vi "GEOM_ReadModifiers.vi"(7 "database path":path, 8 "error in (no error)":errorcluster, 11 "fpa file":path) -> (0 "error out":errorcluster, 2 "modifiers":T2={"Binning"={"x"=1, "y"=1}, "sections"=[]} {"Binning"."y" min=1; "Binning"."x" min=1})   [LabVIEW 2016]
uses:
  GEOM_AmpModifiers.ctl
  GEOM_Binning.ctl
  GEOM_Moifier.ctl
  <vilib>/Utility/config.llb/Read Key (String).vi
  <vilib>/Utility/config.llb/NI_LVConfig.lvlib
panel:
  in  "section":T1
  out "stripped path":path
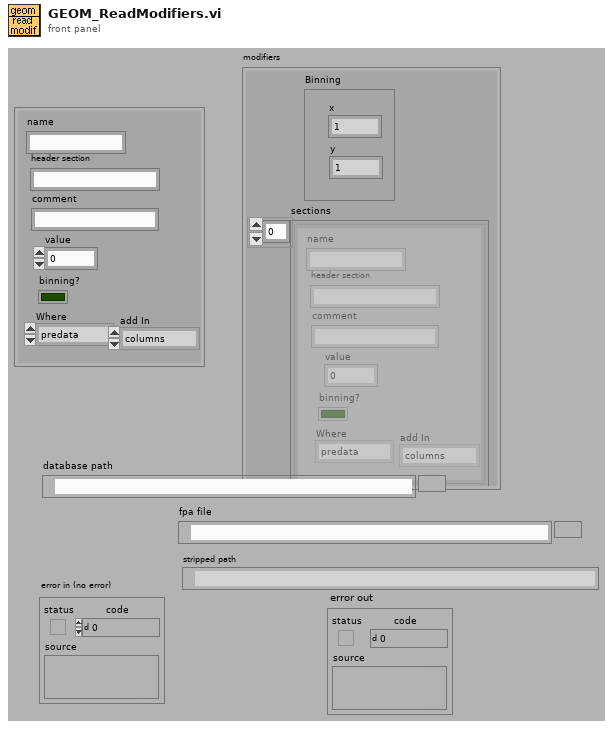
[diagram p1: front panel]
types:
  T1 = cluster{"name":string, "header section":string, "comment":string, "value":i32, "binning?":bool, "Where":enum16{"predata", "postdata"}, "add In":enum16{"columns", "rows", "none"}}
  T2 = typedef "GEOM_AmpModifiers.ctl" = cluster{"Binning":T3, "sections":T4[]}
  T3 = typedef "GEOM_Binning.ctl" = cluster{"x":u32, "y":u32}
  T4 = typedef "GEOM_Moifier.ctl" = cluster{"name":string, "header section":string, "comment":string, "value":i32, "binning?":bool, "Where":enum16{"predata", "postdata"}, "add In":enum16{"columns", "rows", "none"}}
  T5 = cluster{"name":string, "header section":string, "comment":string, "value":i32, "binning?":bool, "Where":enum16{"predata", "postdata"}, "add In":enum16{"columns", "rows", "none"}}[]
  T6 = typedef "NI_LVConfig.lvlib/Config Data RefNum.ctl" = refnum<k1>
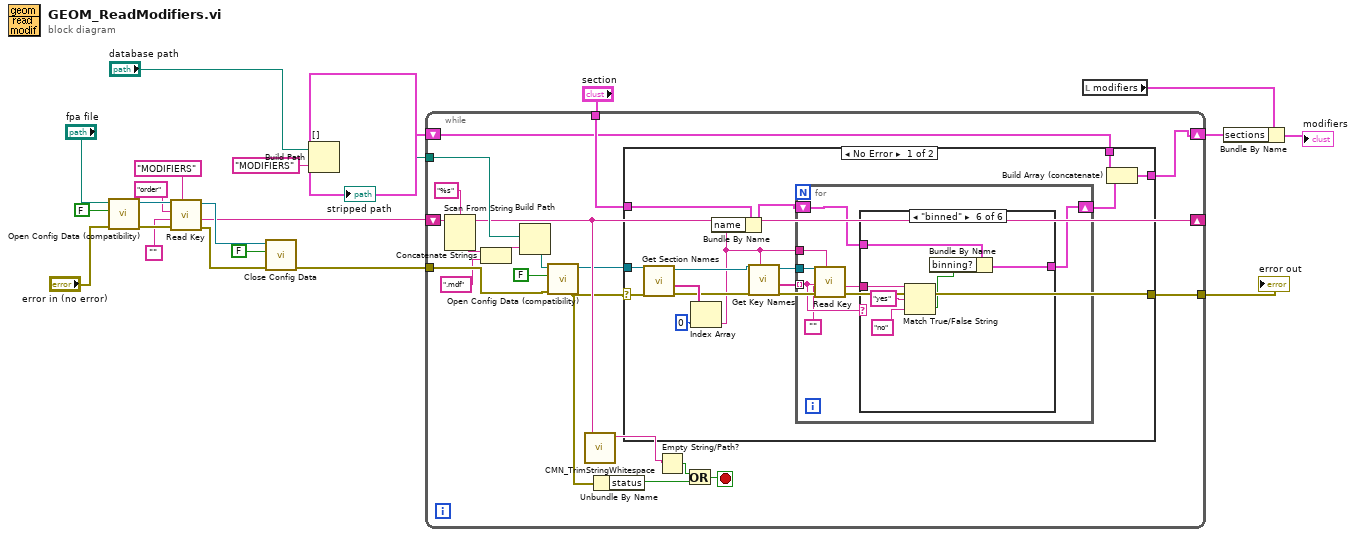
[diagram p0: block diagram]
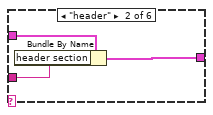
[diagram p3: hidden frame]
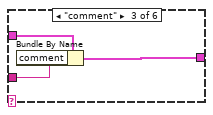
[diagram p4: hidden frame]
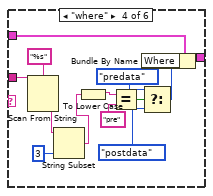
[diagram p5: hidden frame]
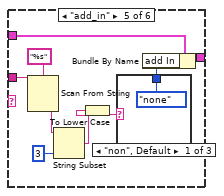
[diagram p6: hidden frame]
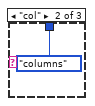
[diagram p7: hidden frame]
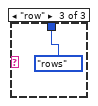
[diagram p8: hidden frame]
diagram:
  n1 = call <vilib>:"Open Config Data (compatibility).vi"("error in (no error)"="error in (no error)", "create file if necessary (T)"=FALSE ("create file if necessary? (T)"), "configuration file path"="fpa file") -> ("error out"=w22:errorcluster, "refnum"=w21:T6)  [unwired: 6 in, 1 out]
  n2 = call-poly <vilib>:"Read Key.vi"("section"="MODIFIERS", "error in (no error)"=w22, "default value"="", "key"="order", "refnum"=w21) -> ("error out"=w16:errorcluster, "value"=w12:string, "refnum out"=w17:T6)  [unwired: 1 in, 3 out]
  n3 = call <vilib>:"Close Config Data.vi"("error in (no error)"=w16, "write file if changed (T)"=FALSE ("write configuration file? (T)"), "refnum"=w17) -> ("error out"=w4:errorcluster)  [unwired: 8 out]
  n4 = Build Path(base path="database path", name or relative path="MODIFIERS") -> (appended path=w11:path)
  "stripped path" <- w11
  n5 = while {
    shift-right: [w37] -> _
    shift-left: w12 -> [w42]
    tunnel: w11 -> [w40]
    tunnel: "section" -> [w31]
    shift-right: [w30] -> w8
    shift-left: T5 [] -> [w29]
    tunnel: w4 -> [w27]
    tunnel: [w26] -> w3
    stop <- w34 stop-if-true
    n6 = Scan From String(format string="%s", input string=w42) -> (remaining string=w37:string, output 1=w25:string)  [unwired: 2 in, 3 out]
    n7 = Concatenate Strings(w25, ".mdf" ("string")) -> (w23:string)
    n8 = Build Path(base path=w40, name or relative path=w23) -> (appended path=w39:path)
    n9 = call <vilib>:"Open Config Data (compatibility).vi"("error in (no error)"=w27, "create file if necessary (T)"=FALSE ("create file if necessary? (T)"), "configuration file path"=w39) -> ("error out"=w33:errorcluster, "refnum"=w32:T6)  [unwired: 6 in, 1 out]
    n10 = call "CMN_TrimStringWhitespace.vi"("string"=w37) -> ("trimmed string"=w36:string)  [unwired: 1 in, 8 out]
    n11 = Unbundle By Name(w33) -> ("status"=w38:bool)
    n12 = case shown="No Error" w33 {
      selector: w33 -> [w55 w102]
      tunnel: w32 -> [w56 _]
      tunnel: w31 -> [w45 _]
      tunnel: [w48 w103] -> w30
      tunnel: w29 -> [w47 w103]
      tunnel: [w46 w102] -> w26
      frame No Error {
        n13 = call <vilib>:"Get Section Names.vi"("error in (no error)"=w55, "refnum"=w56) -> ("error out"=w46:errorcluster, "section names"=w54:string[], "refnum out"=w52:T6)  [unwired: 7 out]
        n14 = Index Array(array=w54, index=0) -> (element=w43:string)
        n15 = Bundle By Name(cluster=w45, "name"=w43) -> (w44:T1)
        n16 = call <vilib>:"Get Key Names.vi"("section"=w43, "refnum"=w52) -> ("key names"=w51:string[], "refnum out"=w50:T6)  [unwired: 1 in, 7 out]
        n17 = for {
          tunnel: w51 -> [w61] mode=indexing
          tunnel: w50 -> [w63]
          tunnel: w43 -> [w62]
          shift-right: [w58] -> w49
          shift-left: w44 -> [w57]
          n18 = call-poly <vilib>:"Read Key.vi"("section"=w62, "default value"="", "key"=w61, "refnum"=w63) -> ("value"=w59:string)  [unwired: 2 in, 5 out]
          n19 = case shown="\"binned\"" w61 {
            tunnel: w57 -> [w64 w67 w70 w83 w92 w101]
            tunnel: w59 -> [_ w66 w69 w76 w90 w99]
            tunnel: [w64 w65 w68 w82 w91 w100] -> w58
            frame Default {
            }
            frame "header" {
              n20 = Bundle By Name(cluster=w67, "header section"=w66) -> (w65:T1)
            }
            frame "comment" {
              n21 = Bundle By Name(cluster=w70, "comment"=w69) -> (w68:T1)
            }
            frame "where" {
              n22 = Scan From String(format string="%s", input string=w76) -> (output 1=w74:string)  [unwired: 2 in, 4 out]
              n23 = String Subset(string=w74, length (rest)=3 ("length (rest)")) -> (substring=w72:string)  [unwired: 1 out]
              n24 = To Lower Case(string=w72) -> (all lower case string=w71:string)
              n25 = Equal?(x=w71, y="pre") -> (x = y?=w80:bool)
              n26 = Select(t=enum16{"predata", "postdata"}."predata" ("Value"), s=w80, f=enum16{"predata", "postdata"}."postdata" ("Value")) -> (s? t:f=w78:enum16{"predata", "postdata"})
              n27 = Bundle By Name(cluster=w83, "Where"=w78) -> (w82:T1)
            }
            frame "add_in" {
              n28 = Scan From String(format string="%s", input string=w90) -> (output 1=w88:string)  [unwired: 2 in, 4 out]
              n29 = String Subset(string=w88, length (rest)=3 ("length (rest)")) -> (substring=w86:string)  [unwired: 1 out]
              n30 = To Lower Case(string=w86) -> (all lower case string=w85:string)
              n31 = case shown="\"non\", Default" w85 {
                tunnel: [enum16{"columns", "rows", "none"}."none" ("Value") enum16{"columns", "rows", "none"}."columns" ("Value") enum16{"columns", "rows", "none"}."rows" ("Value")] -> w84
                frame "non", Default {
                }
                frame "col" {
                }
                frame "row" {
                }
              }
              n32 = Bundle By Name(cluster=w92, "add In"=w84) -> (w91:T1)
            }
            frame "binned" {
              n33 = Match True/False String(2:"no" ("false string"), 3:"yes" ("true string"), 4:w99) -> (0:w96:bool)  [unwired: 1 out]
              n34 = Bundle By Name(cluster=w101, "binning?"=w96) -> (w100:T1)
            }
          }
        }
        n35 = Build Array (concatenate)(w47, w49) -> (w48:T5)
      }
      frame Error {
      }
    }
    n36 = Empty String/Path?(string/path=w36) -> (empty?=w35:bool)
    n37 = Or(x=w35, y=w38) -> (x .or. y?=w34:bool)
  }
  "error out" <- w3
  n38 = local read "modifiers"() -> (w6:T2)
  n39 = Bundle By Name(cluster=w6, "sections"=w8) -> (→"modifiers":T2)
